vi "Generate all possible ABORT addresses.vi"(8 "error in (no error)":errorcluster) -> (0 "error out":errorcluster, 3 "Array":string[](array[string]))   [LabVIEW 2020, in "TALOS.lvlib" / "Guardian.lvlib" / "Guardian.lvclass"]
uses:
  Guardian.lvclass
  Ancestor/Ancestor/Ancestor.lvclass/Ancestor.ctl
  Support VIs/Circus Config Param - Core.vi
  Support VIs/Generate Error.vi
  Support VIs/Circus Root Path.vi
  Support VIs/TALOS Config Param.vi
  FGV/Error Memory/Get Error Description.vi
  Support VIs/Get PC name.vi
  Ancestor/Ancestor/Read ID.vi
  Support VIs/Get Class Name.vi
  <vilib>/Utility/error.llb/Clear Errors.vi
  FGV/Error Memory/Error Memory Core.vi
  <vilib>/AdvancedString/Delimited String to 1D String Array.vi
  FGV/Error Memory/Error Crt Lvl checker.vi
  FGV/Error Memory/Error Memory Core.vi/40c8088d-b597-4017-91af-faa98e00292e.vi
  FGV/Error Memory/Error Memory Core.vi/d4a3ab98-063c-4e44-b43d-fbdcfe6c2be2.vi
  Support VIs/Global Constants.vi
  Support VIs/Global Memory.vi
  <vilib>/Utility/LVClass/Get LV Class Name.vi
  Support VIs/Is in Packed Library.vi
  Support VIs/TALOS Root path.vi
  Support VIs/Read CSV worksheet.vi
  <vilib>/Utility/error.llb/General Error Handler.vi
  <vilib>/Utility/config.llb/Open Config Data.vi
  <vilib>/Utility/config.llb/Get Section Names.vi
  <vilib>/Utility/config.llb/Get Key Names.vi
  <vilib>/Utility/config.llb/Read Key.vi
  <vilib>/Utility/config.llb/Read Key (String).vi
  <vilib>/Utility/config.llb/Close Config Data.vi
  Extract list from Project INI file entry.vi
  Ancestor/Ancestor/Ancestor.lvclass
  <vilib>/Comparison/Equal/Equal Functor/Equal Functor.lvclass
  Guardian.lvclass/Guardian.ctl
  TALOS.lvlib
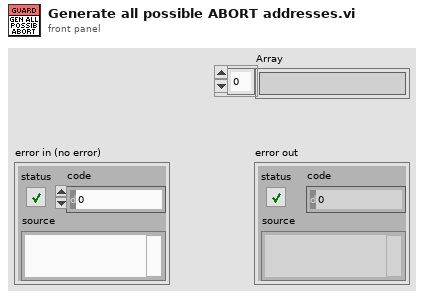
[diagram p1: front panel]
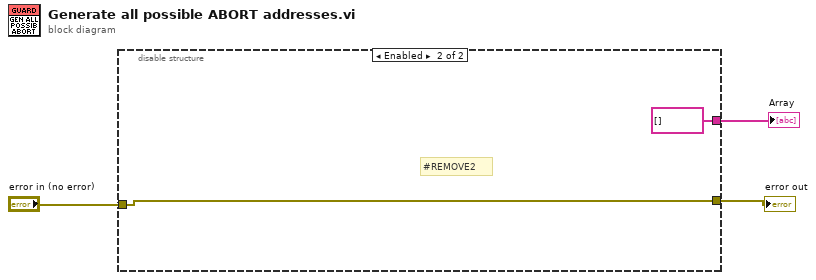
[diagram p0: block diagram]
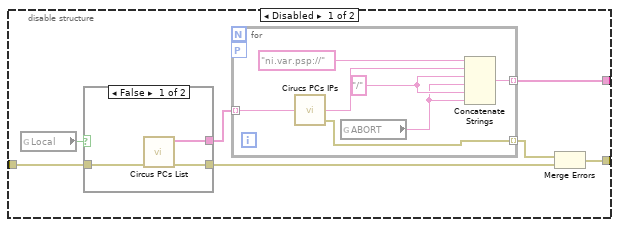
[diagram p2: hidden frame]
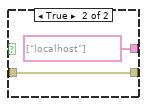
[diagram p3: hidden frame]
diagram:
  n1 = disable-structure shown="Enabled" {
    disable-tunnel: [w9 string[] [] ("Array")] -> w3
    disable-tunnel: "error in (no error)" -> [w8 w23]
    disable-tunnel: [w5 w23] -> w1
    frame Disabled {
      n2 = global read "Global Constants.vi" "Local"() -> (w6:bool)
      n3 = case shown="False" w6 {
        tunnel: [w13 string[] ["localhost"] ("PC List out")] -> w10
        tunnel: w8 -> [w12 w15]
        tunnel: [w11 w15] -> w7
        frame False {
          n4 = call "Circus PCs List.vi"("error in (no error)"=w12) -> ("error out"=w11:errorcluster, "PC List out"=w13:string[])  [unwired: 9 in]
        }
        frame True {
        }
      }
      n5 = for {
        tunnel: w10 -> [w22] mode=indexing
        tunnel: [w17] -> w9 mode=indexing
        workers-P: _ -> [_]
        tunnel: [w16] -> w4 mode=indexing
        w19 = "/" ("string")
        n6 = call "Cirucs PCs IPs.vi"("ID"=w22) -> ("error out"=w16:errorcluster, "IP"=w20:string)  [unwired: 3 in]
        n7 = global read "Global Constants.vi" "ABORT"() -> (w18:string)
        n8 = Concatenate Strings("ni.var.psp://", w20, w19, w18, w19, w18) -> (w17:string)
      }
      n9 = Merge Errors(w4, w7) -> (w5:errorcluster)
    }
    frame Enabled {
      # "#REMOVE2"
    }
  }
  "Array" <- w3
  "error out" <- w1
